vi "_PC_Daemon_Chromatogram.vi"() -> (0 "error out":errorcluster)   [LabVIEW 2018]
uses:
  Chromatogram/DataXControl/DataGraphXControl.xctl
panel:
  in  "BackBtn":bool
  in  "Document Path":path
  in  "Loaded Voltage":bool
  in  "Document Tree":string[](tree)=["D:\\ATI_MS_InstrumentControl_08_08_00\\MSData\\Untitled.list"]
  in  "XICGraph":T1(xcontrol)
  in  "MassGraph":T1(xcontrol)
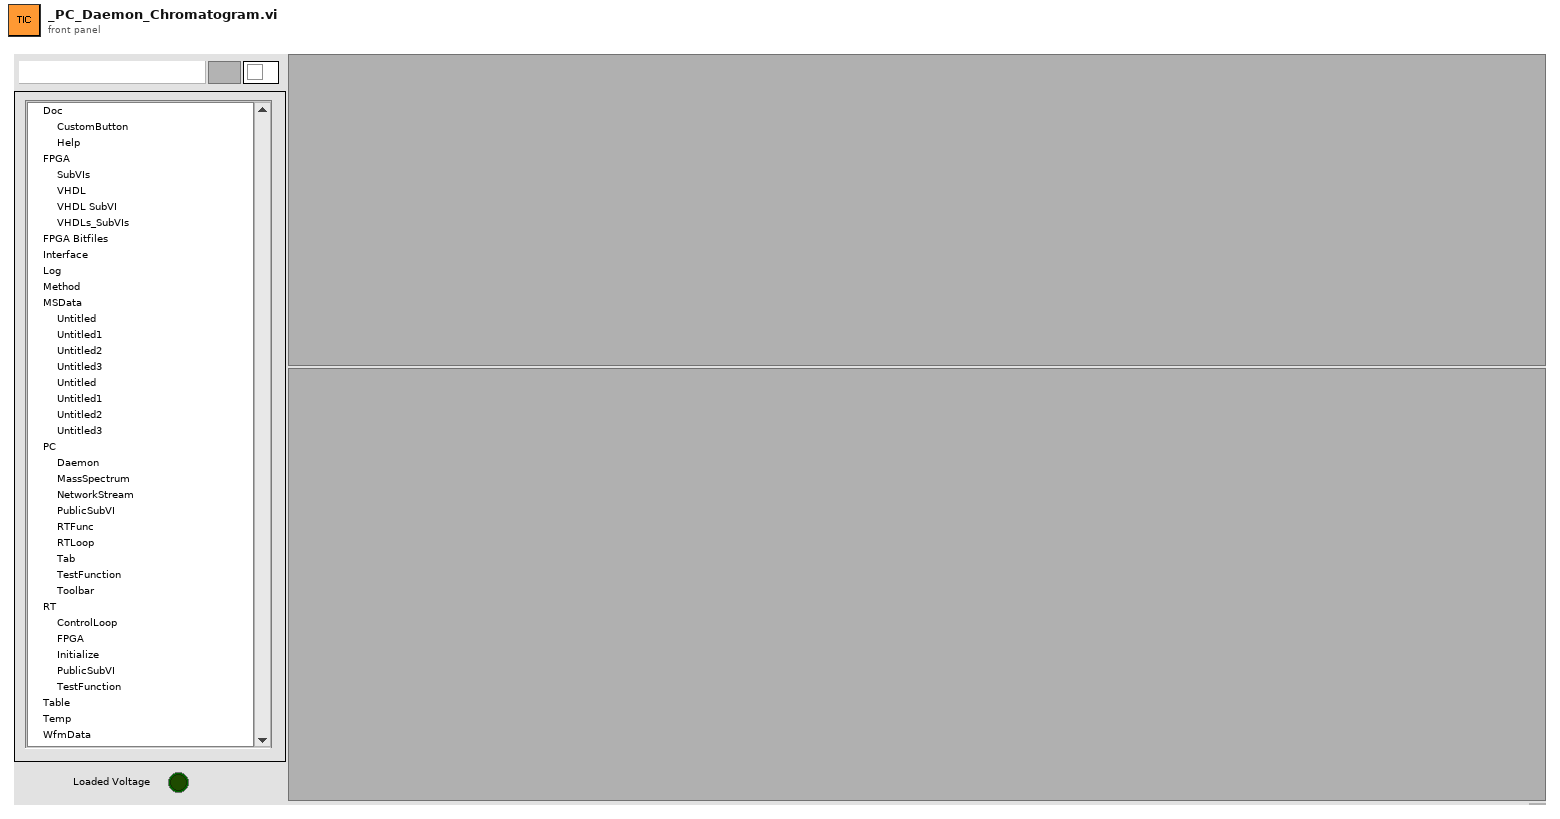
[diagram p1: front panel]
types:
  T1 = cluster{"FilePath":path, "Data State":enum16{"Mass", "XIC"}, "Data Plot Names":string[], "DataArray":cluster{"X":dbl[], "Y":dbl[]}[], "Volt Plot Names":string[], "VoltArray":cluster{"X":dbl[], "Y":dbl[]}[], "UserDefine":cluster{"Label":string, "Variant":variant}, "Information":variant}
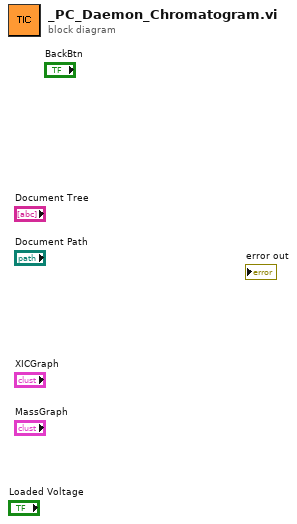
[diagram p0: block diagram]
diagram:
